vi "Write Address.vi"(8 "error in (no error)":errorcluster, 10 "Address":string, 11 "Alicat Device in":refnum<class "Alicat Device.lvclass">) -> (0 "error out":errorcluster, 3 "Alicat Device out":refnum<class "Alicat Device.lvclass">)   [LabVIEW 2018, in "Alicat Lib.lvlib" / "Alicat Device.lvclass"]
uses:
  Alicat Device.lvclass
  C:/Users/Labview/Documents/exscalabar_server/Devices/Configurable Device/Configurable Device.lvclass
  Configurable Device/Configurable Device.lvclass/Configurable Device.ctl
  Alicat Device.lvclass/Alicat Device.ctl
  Configurable Device/Accessors/Write Addr.vi
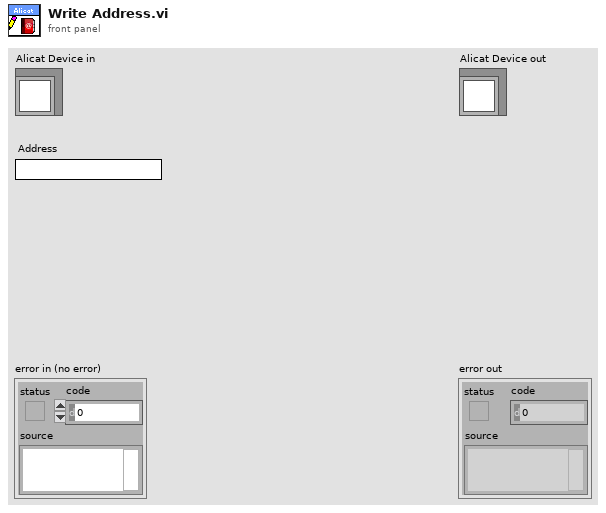
[diagram p1: front panel]
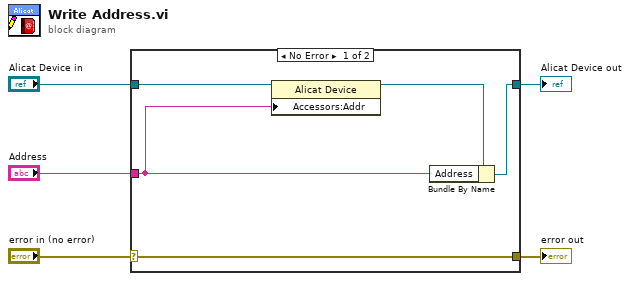
[diagram p0: block diagram]
diagram:
  n1 = case shown="No Error" "error in (no error)" {
    selector: "error in (no error)" -> [w10 w11]
    tunnel: [w10 w11] -> w4
    tunnel: [w9 w12] -> w2
    tunnel: "Alicat Device in" -> [w8 w12]
    tunnel: "Address" -> [w6 _]
    frame No Error {
      n2 = property class="Alicat Device"(reference=w8, "Accessors:Addr"=w6) -> (reference out=w7:refnum<class "Alicat Device.lvclass">)  [unwired: 1 in, 1 out]
      n3 = Bundle By Name(cluster=w7, "Address"=w6) -> (w9:refnum<class "Alicat Device.lvclass">)
    }
    frame Error {
    }
  }
  "error out" <- w4
  "Alicat Device out" <- w2
